vi "PRL BUFFER Cut from Analog 2D Array.vi"(9 "Cut Index":i32, 10 "Signal Index":i32, 11 "Array In":sgl[][](array[numeric])) -> (3 "Array Out":sgl[](array[numeric]))   [LabVIEW 2013, in "PMU Recorder Light.lvlib"]
uses:
  PMU Recorder Light.lvlib
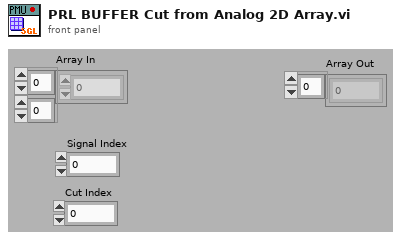
[diagram p1: front panel]
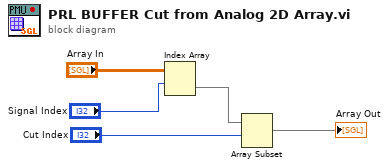
[diagram p0: block diagram]
diagram:
  n1 = Index Array(array="Array In", index (row)="Signal Index") -> (element=w3:sgl[])  [unwired: 1 in]
  n2 = Array Subset(array=w3, index="Cut Index") -> (→"Array Out":sgl[])  [unwired: 1 in]
